vi "SteuerungWaermepumpe-altes FrontPanel_31.01.2017.vi"() -> ()   [LabVIEW 2015]
uses:
  <vilib>/DAQmx/read.llb/DAQmx Read (Analog 1D Wfm NChan NSamp).vi
  <vilib>/DAQmx/write.llb/DAQmx Write (Analog 1D Wfm NChan 1Samp).vi
  <vilib>/MakerHub/LINX/Public/Peripherals/Digital/Digital Write N Chans.vi
  <vilib>/MakerHub/LINX/Private/Local IO/LinxDigitalWrite.vi
  <vilib>/MakerHub/LINX/Public/Utilities/Check Channel.vi
  <vilib>/MakerHub/LINX/Private/Utilties/Generate Error.vi
  <vilib>/DAQmx/miscellaneous.llb/DAQmx Fill In Error Info.vi
  <vilib>/Utility/file.llb/Read Delimited Spreadsheet (DBL).vi
  <vilib>/MakerHub/LINX/LMH-LINX.lvlib
panel:
  in  "Keithley Messung?":bool
  in  "TI 21a SW °C":dbl=60.0 min=30.0 max=60.0
  in  "Öl-Regelung":bool
  out "Array 2":waveform(dbl)[](array[waveform])
  in  "Wartezeit 2":u32=500
  in  "Wartezeit 1":u32=9000
  out "Abscheider":cluster{dbl, dbl, dbl}(slide) scale=0.0..1.3
  in  "Rampe":bool=TRUE
  in  "Rampe rpm/s":dbl=1.0 min=1.0 max=100.0 step=1.0
  out "Rampe IW":dbl
  in  "reinitialize HD":bool
  in  "reinitialize Pumpe":bool
  out "ist an!":string
  in  "zusätzlicher Druck":dbl
  in  "PI05 SW":dbl format="%.2f"
  out "p_liq_mittel":dbl
  out "p_liq":dbl
  out "Schleifendauer":dbl format="%.5f"
  out "Mittelwert 2":dbl
  in  "Mittelwert HD":bool
  in  "Mittelwert Pumpe":bool
  out "Mittelwert":dbl
  in  "Xi / p_liq berechnung an":bool
  out "xi_r":dbl
  in  "Regler Senke":bool
  in  "reinitialize Senke":bool
  in  "TI35 SW":dbl=43.0 format="%.2f"
  in  "Drehzahl Bestätigung":bool
  in  "Drehzahl SW":dbl=1000.0 min=500.0 max=3000.0 step=1.0 format="%#_4g"
  out "Check":dbl format="%#_13g"
  in  "Regler Hochdruck":bool
  in  "PID Regelung Pumpe":bool
  in  "SW TI39":dbl
  out "Array":bool[](array[boolean])
  in  "LEDs 2":bool[](array[boolean])
  in  "Regelung HK":bool
  out "RV 30 zu":bool
  out "RV 30 auf":bool
  out "FI_Oel":dbl
  in  "RV 33":dbl(slide) scale=-1.0..1.0
  in  "tag":string
  out "Pumpenwerte":dbl[](array[numeric]) format="%.2f"
  out "Speichert!":bool
  out "Historie":string
  in  "Kommentar":string
  out "refnum out":refnum<file>
  in  "Identität!":string(combo)
  in  "Zeit X in Minuten":dbl(slide)=5.0 min=0.0 max=15.0 scale=5.0..15.0
  out "TI 21a Warnungen":dbl
  out "Leistung":dynamicdata(graph)
  out "TI 37":dbl
  in  "Programm stoppen!":bool
  out "%":sgl(slide) scale=0.0..100.0
  out "kalt":bool
  out "warm":bool
  out "?":T1(array[cluster]) {"?" format="%#.4g"; "Konzentration_reich" format="%#.4g"}
  in  "Mit EES vergleichen":bool
  in  "FI13 SW in l/min":dbl=3.0 min=3.0 max=20.0 step=0.10000000149011612
  out "COP_Oel":dbl
  out "Q-Oel kW":dbl format="%_4g"
  in  "Dateiname!":string
  in  "Comment":bool
  in  "Speichern":bool caption="Aktivieren"
  out "ZU     Ventilstellung 33     AUF":dbl(slide) scale=0.0..100.0 scale format="%.2f"
  in  "Regelventil 34":dbl(slide) min=0.0 max=100.0 step=0.009999999776482582 scale=0.0..100.0
  in  "Matlab":bool
  in  "?":T2(tab)
  out "?":dynamicdata(graph)
  out "?":waveform(dbl)(graph)
  out "?":dynamicdata(graph)
  out "PI 12":dbl format="%.2f"
  out "PI 11":dbl format="%.2f"
  out "Dichte":dbl format="%.5g"
  in  "Reset":bool
  out "Betriebszeit":cluster{"second":i32, "minute":i32, "hour":i32}
  out "Temperatur Ölprüfstand":dbl
  out "FI 13 kg/min":dbl
  in  "Messung\nFrequenzwandler":bool
  out "Magnetventil":bool
  out "Fl.Pumpe an":bool
  out "Temperatur Öl":bool
  out "COP":dbl format="%#_13g"
  out "Verdichteraktivität":cluster{"second":i32, "minute":i32, "hour":i32}
  out "Q-Entgaser kW":dbl format="%_4g"
  out "Warnungen":bool[](array[boolean])
  out "Status Komponenten":bool[](array[boolean])
  in  "Pumpen-Auto-Abschalt":bool=TRUE
  out "Q-Resorber kW":dbl format="%_4g"
  out "Stellung Expansionsventil":waveform(dbl)(graph)
  out "FI 35 l/min":dbl format="%#_13g"
  out "FI 38 l/min":dbl format="%#_13g"
  out "FI Oel l/min":dbl format="%#.3g"
  out "LI in l":dbl format="%#_4g"
  out "TI 39":dbl format="%#_3g"
  out "TI 38":dbl format="%#_3g"
  out "TI 36":dbl format="%#_3g"
  out "TI 35":dbl format="%#_3g"
  out "TI 33":dbl format="%#_3g"
  out "TI 32":dbl format="%#_3g"
  out "TI 34":dbl format="%#_3g"
  out "TI 21a":dbl format="%#_3g"
  out "TI 21":dbl format="%#_3g"
  out "TI 20":dbl format="%#_3g"
  out "TI 14a":dbl format="%#_3g"
  out "TI 14":dbl format="%#_3g"
  out "TI 13":dbl format="%#_3g"
  out "TI 12":dbl format="%#_3g"
  out "TI 11":dbl format="%#_3g"
  out "TI 10":dbl format="%#_3g"
  out "TI 09":dbl format="%#_3g"
  out "TI 08":dbl format="%#_3g"
  out "TI 07":dbl format="%#_3g"
  out "TI 06a":dbl format="%#_3g"
  out "TI 06":dbl format="%#_3g"
  out "TI 05":dbl format="%#_3g"
  out "TI 04":dbl format="%#_3g"
  out "TI 22":dbl format="%#_3g"
  out "TI 02":dbl format="%#_3g"
  out "TI 01":dbl format="%#_3g"
  out "Konzentration":dbl format="%#_5g"
  in  "Pumpensteuerung":dbl min=0.0 max=10.0 step=0.009999999776482582 format="%.2g"
  out "PI 08":dbl format="%.2f"
  out "PI 05":dbl format="%#.2f"
  out "PI 02":dbl format="%.2f"
  out "PI 04":dbl format="%.2f"
  out "PDI 8-9":dbl format="%.2f"
  out "PI 14":dbl format="%.2f"
  out "PI 01":dbl format="%.2f"
  out "ZU    Ventilstellung Exp.V     AUF":dbl(slide) scale=0.0..100.0 scale format="%#.1f"
  in  "Exp.V":dbl(slide)=3.0 min=0.0 max=100.0 step=1.0 scale=0.0..100.0 scale format="%#.0f"
  out "ZU    Ventilstellung 14      AUF":dbl(slide) caption="Auf    Ventilstellung 14      Zu" scale=0.0..100.0 scale format="%#.2f"
  in  "Regelventil 36":dbl(slide) min=0.0 max=100.0 step=0.009999999776482582 scale=0.0..100.0 scale format="%#.0f"
  out "ZU  Ventilstellung 35  AUF":dbl(slide) scale=0.0..100.0 scale format="%.2f"
  in  "Regelventil 35":dbl(slide) min=0.0 max=100.0 step=0.009999999776482582 scale=0.0..100.0 scale format="%#.3g"
  out "ZU     Ventilstellung 39     AUF":dbl(slide) scale=0.0..100.0 scale format="%.2f"
  in  "Regelventil 39":dbl(slide)=100.0 min=0.0 max=100.0 step=0.009999999776482582 scale=0.0..100.0
  out "FI 13 l/min":dbl format="%.2f"
  out "FI 07 l/min":dbl format="%.2f"
  out "LI in m":dbl format="%.2f"
  out "PDI 5-6":dbl format="%.4f"
  out "PI 07":dbl format="%.2f"
  out "Druckverhältnis":dbl
  out "Drehzahl":dbl
  out "Drehmoment":dbl
  out "Frequenz":dbl
  out "Leistung":dbl
  out "Durchfluss":waveform(dbl)[](graph)
  in  "Tab Control Temperaturen":T3(tab)
  out "Temperatur Reich":waveform(dbl)[](graph)
  out "Temperatur Arm":waveform(dbl)[](graph)
  out "Temperatur Öl":waveform(dbl)[](graph)
  out "Temperatur Senke/Quelle":waveform(dbl)[](graph)
  out "Druck":waveform(dbl)[](graph)
  out "Druckzustand":bool caption="Zu viel Druck !!!"
  # "Öltemperatur"
  # "Resorber"
  # "Entgaser"
  # "Druckverhältnis"
  # "ExpV"
  # "Verdichter an"
  # "iWÜ"
  # "Magnetventil"
  # "RV 39"
  # "Leer"
  # "RV 33"
  # "RV 35"
  # "RV 34"
  # "Pumpe an"
  # "Ölabscheider"
  # "2"
  # "1"
  # "RV 30"
  # "Verdichter"
  # "Pumpe"
  # "Leistung"
  # "kW"
  # "Speed"
  # "rpm"
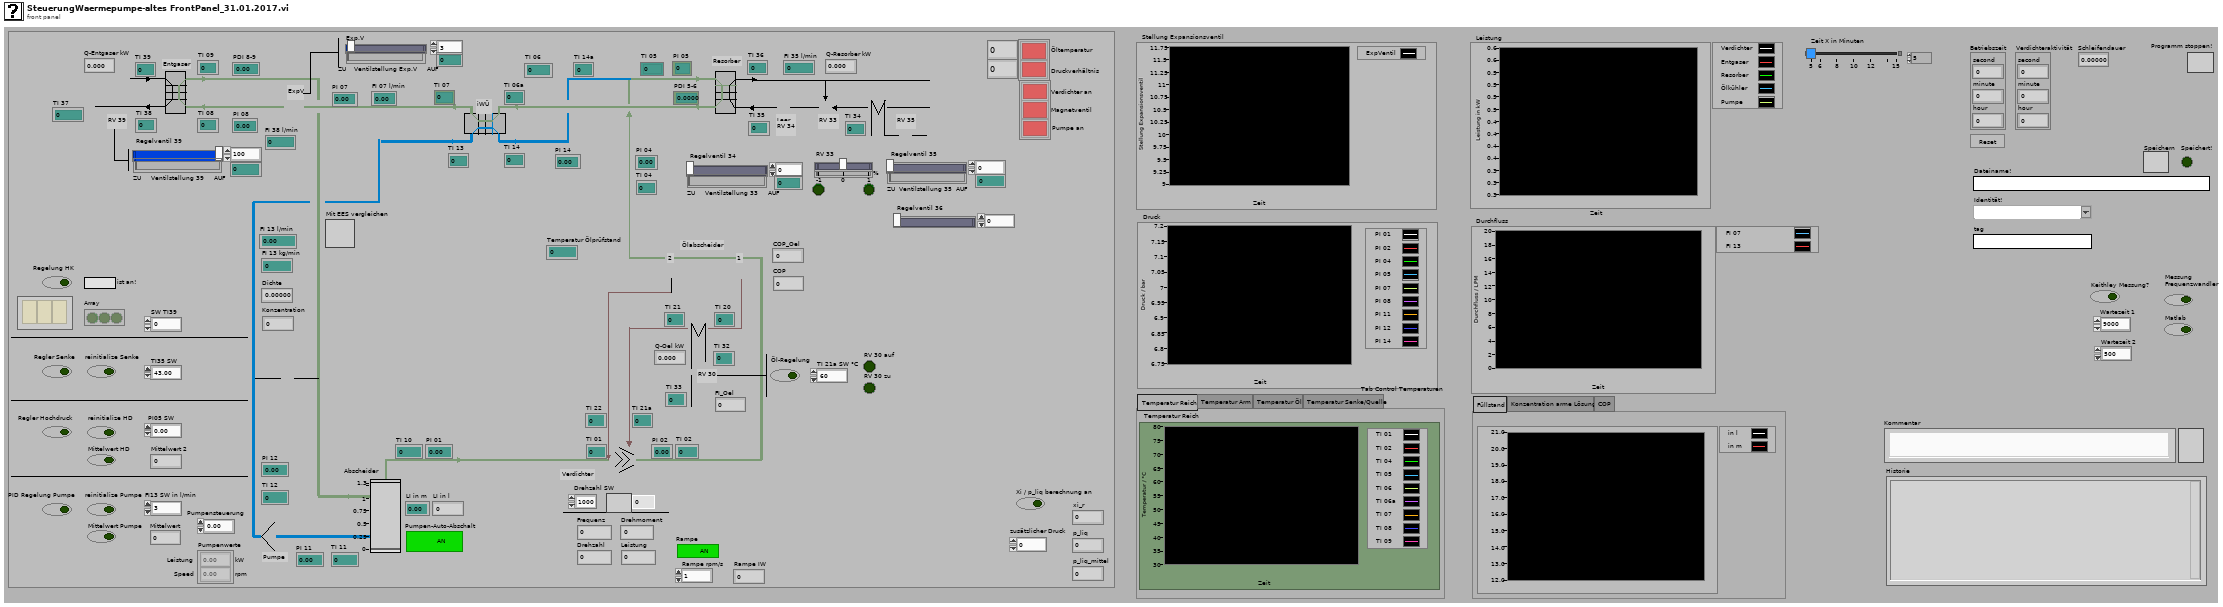
[diagram p1: front panel]
types:
  T1 = cluster{dbl, "Konzentration_reich":dbl, "String":string, bool}[]
  T2 = enum32{"Füllstand", "Konzentration arme Lösung", "COP"}
  T3 = enum32{"Temperatur Reich", "Temperatur Arm", "Temperatur Öl", "Temperatur Senke/Quelle"}
  T4 = enum8{"Enabled", "Disabled", "Disabled and Grayed Out"}
  T5 = typedef "LMH-LINX.lvlib/LINX Ref.ctl" = cluster{"IO":T6, "Interface":T7, "LINX Device Config":T8}
  T6 = typedef "LMH-LINX.lvlib/Platform.ctl" = enum16{"Remote", "Local"}
  T7 = typedef "LMH-LINX.lvlib/Interface.ctl" = enum16{"Serial", "TCP"}
  T8 = typedef "LMH-LINX.lvlib/Device.lvlib/LINX Device Config.ctl" = cluster{"Interface":T7, "COM Port":refnum<visa-resource-name>, "TCP Configuration":T9, "Device Family":u8, "Device ID":u8, "Device Name":string, "TCP Ref":refnum<k5>, "Channels":T10}
  T9 = typedef "LMH-LINX.lvlib/Device.lvlib/TCP Config.ctl" = cluster{"IP Address":string, "Port":u16}
  T10 = typedef "LMH-LINX.lvlib/Channels.ctl" = cluster{"DI":u8[], "DO":u8[], "AI":u8[], "AO":u8[], "PWM":u8[], "QE":u8[], "UART":u8[], "I2C 2":u8[], "SPI":u8[], "CAN":u8[], "Servo":u8[], "AI Ref (V)":dbl, "AI Resolution (Bits)":u8, "AO Ref (V)":dbl, "AO Resolution (Bits)":u8}
  T11 = enum16{"open", "replace", "create", "open or create", "replace or create", "replace or create with confirmation"}
  T12 = cluster{"Array[0]":dbl, "Array[1]":dbl, "Array[2]":dbl}
  T13 = cluster{"Array[0]":sgl, "Array[1]":sgl, "Array[2]":sgl}
  T14 = cluster{"Numeric":dbl, "Konzentration_reich":dbl, "String":string, bool}[]
  T15 = typedef "LVDateTimeRec.ctl" = cluster{"fractional second":dbl, "second":i32, "minute":i32, "hour":i32, "day of month":i32, "month":i32, "year":i32, "day of week":i32, "day of year":i32, "DST":i32}
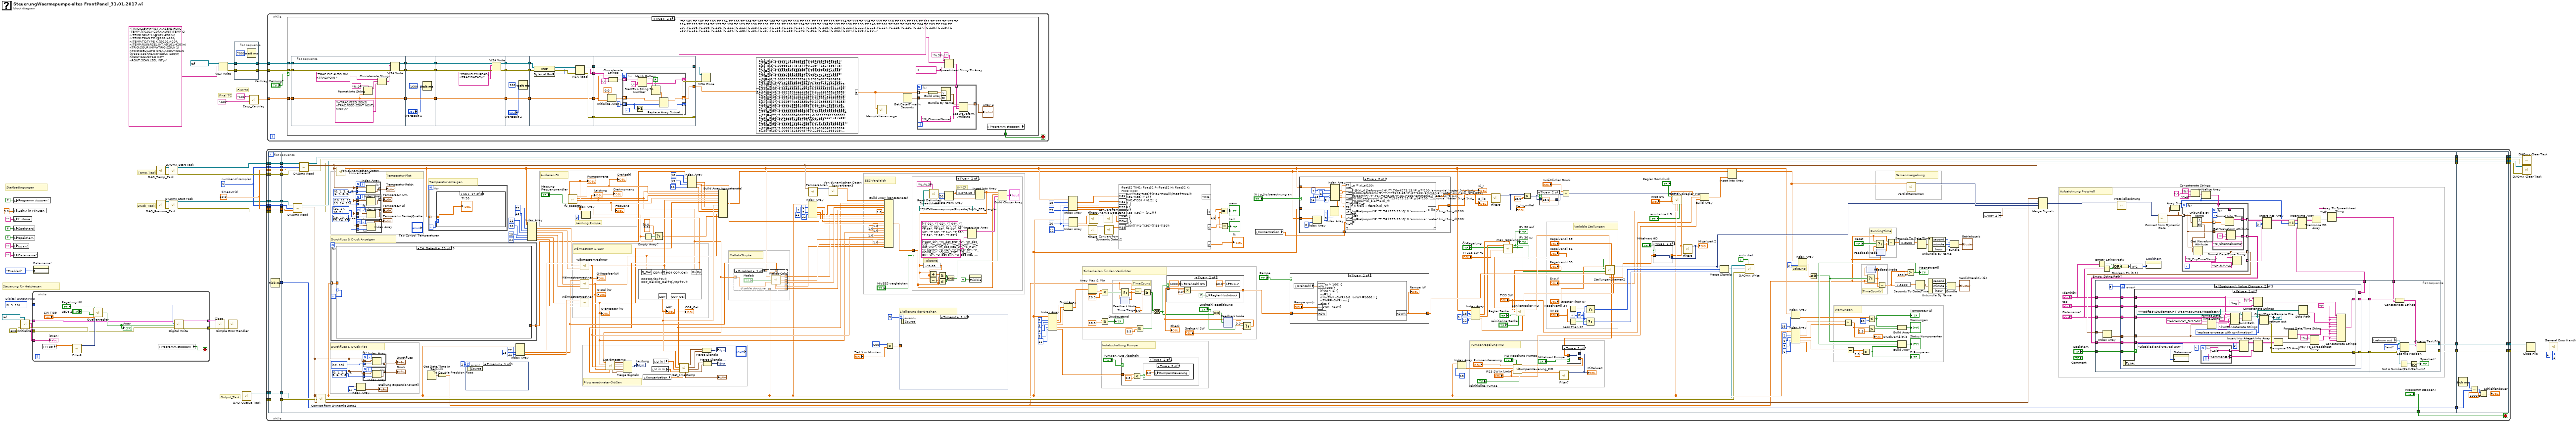
[diagram p0: block diagram]
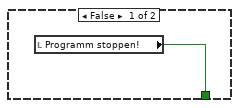
[diagram p2: hidden frame]
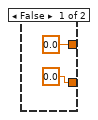
[diagram p8: hidden frame]
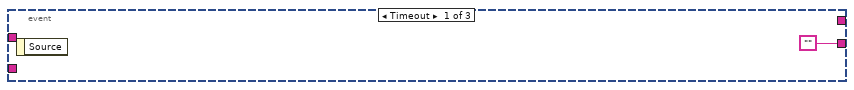
[diagram p10: hidden frame]
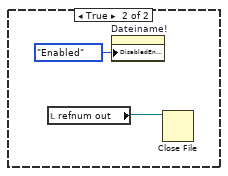
[diagram p11: hidden frame]
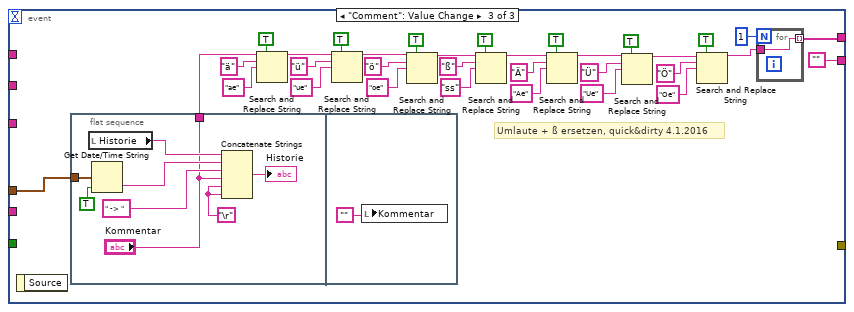
[diagram p12: hidden frame]
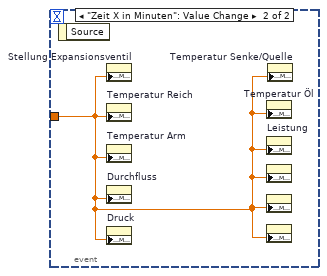
[diagram p13: hidden frame]
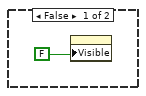
[diagram p14: hidden frame]
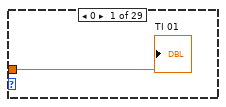
[diagram p17: hidden frame]
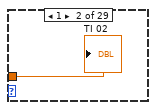
[diagram p18: hidden frame]
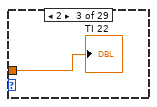
[diagram p19: hidden frame]
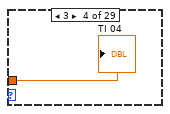
[diagram p20: hidden frame]
diagram:
  w19 = 10.0  # timeout (s)
  w18 = 1  # number of samples
  w31 = i32[] [8, 9, 10]  # Digital Output PIns
  # "Final TC"
  # "First TC"
  # "Output_Task"
  # "Druck_Task"
  # "Temp_Task"
  # "Steuerung für Heizkerzen"
  # "Startbedingungen"
  n1 = local write "Programm stoppen!"(FALSE ("Programm stoppen!")) -> ()
  n2 = local write "Zeit X in Minuten"(5.0 ("Zeit X in Minuten")) -> ()
  n3 = local write "Historie"("") -> ()
  n4 = local write "Speichert!"(FALSE ("Speichert!")) -> ()
  n5 = local write "Speichern"(FALSE ("Speichern")) -> ()
  n6 = local write "ist an!"("") -> ()
  n7 = local write "Dateiname!"("") -> ()
  n8 = call <vilib>:"Initialize.vi"("Serial Port"=refnum<visa-resource-name> "COM4", "Error In"=errorcluster {"status"=FALSE, "code"=0, "source"=""}) -> ("Error Out"=w32:errorcluster, "Device Name"=w29:string, "LINX Resource"=w35:T5)  [unwired: 7 in]
  n9 = while {
    tunnel: w35 -> [w50]
    tunnel: [w60] -> w34
    tunnel: [w59] -> w33
    tunnel: w32 -> [w49]
    tunnel: w31 -> [w58]
    tunnel: w29 -> [w48]
    stop <- w57 stop-if-true
    n10 = local read "TI 39"() -> (w51:dbl)
    n11 = call "Filter6"("Signal"=w51) -> ("Filtered Signal"=w52:dynamicdata)  [unwired: 9 in, 1 out]
    n12 = call "Quellenregler.vi"("Regelung Quelle"="Regelung HK", "TI 38 IW °C"=w52, "LEDs"="LEDs 2", "TI 38 SW °C"="SW TI39") -> ("Kerzen von Regler"=w54:bool[])  [unwired: 3 in, 1 out]
    "Array" <- w54
    n13 = local read "Programm stoppen!"() -> (w57:bool)
    n14 = call-poly <vilib>:"Digital Write.vi"("Error In"=w49, "Values"=w54, "DO Channels"=w58, "LINX Resource"=w50) -> ("Error Out"=w59:errorcluster, "LINX Resource"=w60:T5)  [unwired: 6 in]
    "ist an!" <- w48
  }
  n15 = property on="Dateiname!" class="Str"("DisabledEnum"=T4."Enabled" ("Disabled")) -> ()  [unwired: 2 in, 2 out]
  n16 = call "DAQ_Pressure_Task.vi"() -> ("error out"=w23:errorcluster, "task out"=w24:refnum<k21>)  [unwired: 10 in]
  n17 = call "DAQ_Temp_Task.vi"() -> ("error out"=w25:errorcluster, "task out"=w26:refnum<k21>)  [unwired: 10 in]
  n18 = call <vilib>:"DAQmx Start Task.vi"("task/channels in"=w24, "error in"=w23) -> ("task out"=w17:refnum<k21>, "error out"=w20:errorcluster)  [unwired: 12 in]
  n19 = call <vilib>:"DAQmx Start Task.vi"("task/channels in"=w26, "error in"=w25) -> ("task out"=w21:refnum<k21>, "error out"=w22:errorcluster)  [unwired: 12 in]
  n20 = call <vilib>:"Close.vi"("Error In"=w33, "LINX Resource"=w34) -> ("Error Out"=w36:errorcluster)  [unwired: 9 in]
  n21 = VISA Write(VISA resource name=refnum<visa-resource-name> "COM3", write buffer="TRAC:CLE\n\n*RST\n\nSENS:FUNC 'TEMP',(@101:420)\n\nUNIT:TEMP C\n:TEMP:NPLC 1,(@101:420)\n\n:TEMP:TRAN TC,(@101:420)\n:TEMP:TC:TYPE K,(@101:420)\n:TEMP:RJUN:RSEL INT,(@101:420)\n\nTRIG:SOUR IMM\nTRIG:COUN 1\nTRIG:DEL:AUTO ON\n\nROUT:SCAN  (@101:420)\nSAMP:COUN 120\n\nROUT:SCAN:TSO IMM\nROUT:SCAN:LSEL INT\n") -> (VISA resource name out=w5:refnum<visa-resource-name>, error out=w6:errorcluster)  [unwired: 1 in, 1 out]
  n22 = call <vilib>:"Simple Error Handler.vi"("error in (no error)"=w36) -> ()  [unwired: 4 in, 5 out]
  n23 = flat-sequence {
    tunnel: w6 -> [w63]
    tunnel: [w63] -> w3
    tunnel: w5 -> [w61]
    tunnel: [w61] -> w4
    frame #0 {
      n24 = Wait (ms)(milliseconds to wait=u32 7000 ("Zu wartende ms")) -> ()  [unwired: 1 out]
    }
  }
  n25 = call "DAQ_Output_Task.vi"() -> ("error out"=w11:errorcluster, "task out"=w12:refnum<k21>)  [unwired: 10 in]
  n26 = call "Easy_Keithley.vi"("Final Thermocouple ID# (String)"="420", "First Thermocouple ID# (String)"="101") -> ("Number of Thermocouples"=w7:dbl)  [unwired: 8 in, 1 out]
  n27 = while {
    tunnel: [w98] -> w41
    tunnel: [w97] -> w40
    tunnel: w22 -> [w91]
    tunnel: w19 -> [w89]
    tunnel: w21 -> [w86]
    tunnel: w18 -> [w84]
    tunnel: w20 -> [w82]
    tunnel: w19 -> [w81]
    tunnel: w18 -> [w79]
    tunnel: w17 -> [w77]
    tunnel: [w73] -> w16
    tunnel: [w72] -> w15
    tunnel: [w70] -> w14
    tunnel: [w68] -> w13
    tunnel: w12 -> [w67]
    tunnel: w11 -> [w64]
    stop <- w96 stop-if-true
    n28 = flat-sequence {
      tunnel: [w109] -> w92
      tunnel: w91 -> [w108]
      tunnel: [w108] -> w90
      tunnel: w89 -> [w107]
      tunnel: [w107] -> w88
      tunnel: w86 -> [w106]
      tunnel: [w106] -> w87
      tunnel: [w105] -> w85
      tunnel: w84 -> [w105]
      tunnel: [w104] -> w83
      tunnel: w82 -> [w104]
      tunnel: w81 -> [w103]
      tunnel: [w103] -> w80
      tunnel: w79 -> [w102]
      tunnel: [w102] -> w78
      tunnel: w77 -> [w101]
      tunnel: [w101] -> w76
      tunnel: w67 -> [w100]
      tunnel: [w100] -> w66
      tunnel: [w99] -> w65
      tunnel: w64 -> [w99]
      tunnel: ["Programm stoppen!"] -> w96
      tunnel: [w333] -> w95
      tunnel: [w332] -> w94
      tunnel: [w141] -> w93
      tunnel: w92 -> [w141]
      tunnel: w90 -> [w176]
      tunnel: w88 -> [w175]
      tunnel: w87 -> [w174]
      tunnel: w85 -> [w173]
      tunnel: w83 -> [w172]
      tunnel: w80 -> [w171]
      tunnel: w78 -> [w170]
      tunnel: w76 -> [w169]
      tunnel: [w168] -> w75
      tunnel: [w167] -> w74
      tunnel: [w166] -> w71
      tunnel: [w165] -> w69
      tunnel: w66 -> [w163]
      tunnel: w65 -> [w162]
      tunnel: [w742] -> w97
      tunnel: [w743] -> w98
      tunnel: w95 -> [w743]
      tunnel: w94 -> [w742]
      tunnel: w93 -> [w740]
      tunnel: w75 -> [w735]
      tunnel: w74 -> [w736]
      tunnel: [w736] -> w73
      tunnel: [w735] -> w72
      tunnel: w71 -> [w734]
      tunnel: [w734] -> w70
      tunnel: w69 -> [w733]
      tunnel: [w733] -> w68
      frame #0 {
        n29 = Tick Count (ms)() -> (millisecond timer value=w109:u32)
      }
      frame #1 {
        w143 = 8.0  # Time Target
        w164 = TRUE  # auto start
        w353 = sgl 1.0
        w366 = 22
        w371 = 20
        w397 = -4
        w398 = 0
        # "RunningTime"
        # "TimeCountV"
        # "TimeCount"
        # "Sicherheiten für den Verdichter"
        # "Pumpenregelung PID"
        # "Skalierung der Graphen"
        # "Leistung Pumpe"
        # "Leistung"
        # "Durchfluss & Druck Anzeigen"
        # "Temperatur Anzeigen"
        # "Plots errechneter Größen"
        # "EES-Vergleich"
        # "Matlab-Skripte"
        # "Warnungen"
        # "Namensvergebung"
        # "Wärmestrom & COP"
        # "Notabschaltung Pumpe"
        # "Auslesen FU"
        # "Durchfluss & Druck Plot"
        # "Temperatur Plot"
        # "Aufzeichnung Protokoll"
        # "Variable Stellungen"
        n30 = call-poly <vilib>:"DAQmx Read.vi"("task/channels in"=w169, "number of samples per channel"=w170, "timeout"=w171, "error in"=w172) -> ("task out"=w168:refnum<k21>, "data"=w178:waveform(dbl)[], "error out"=w165:errorcluster)  [unwired: 9 in]
        n31 = call-poly <vilib>:"DAQmx Read.vi"("task/channels in"=w174, "number of samples per channel"=w173, "timeout"=w175, "error in"=w176) -> ("task out"=w167:refnum<k21>, "data"=w177:waveform(dbl)[], "error out"=w166:errorcluster)  [unwired: 9 in]
        n32 = call "Convert from Dynamic Data2"("Dynamic Data Type"=w178) -> ("Array"=w183:dbl[])  [unwired: 3 in]
        n33 = for {
          tunnel: w183 -> [w681] mode=indexing
          tunnel: [w680] -> w188 mode=indexing
          i -> [w682]
          n34 = case shown="24, Default" w682 {
            tunnel: w681 -> [w683 w684 w685 w686 w687 w688 w689 w690 w691 w692 w693 w702 w714 w717 w718 w719 w720 w721 w724 w728 w729 w730 w731 w732 _]
            tunnel: [_ _ _ _ _ _ _ _ _ _ _ w694 _ _ _ _ _ _ w722 w726 _ _ _ _ _] -> w680
            frame 0 {
              "PI 01" <- w683
            }
            frame 1 {
              "PI 02" <- w684
            }
            frame 2 {
              "PI 04" <- w685
            }
            frame 3 {
              "PI 05" <- w686
            }
            frame 4 {
              "PI 07" <- w687
            }
            frame 5 {
              "PI 08" <- w688
            }
            frame 6 {
              "PI 11" <- w689
            }
            frame 7 {
              "PI 12" <- w690
            }
            frame 8 {
              "PI 14" <- w691
            }
            frame 9 {
              "PDI 5-6" <- w692
            }
            frame 10 {
              "PDI 8-9" <- w693
            }
            frame 11 {
              n35 = call "Filter3"("Signal"=w702) -> ("Filtered Signal"=w700:dynamicdata)  [unwired: 9 in, 1 out]
              n36 = Greater?(x=w702, y=0.3) -> (0:w697:bool)
              n37 = case shown="False" w697 {
                tunnel: w702 -> [_ w713]
                tunnel: [0.0 w713] -> w705
                frame False {
                }
                frame True {
                }
              }
              n38 = call "Convert from Dynamic Data6"("Dynamic Data Type"=w700) -> ("Scalar"=w699:dbl)  [unwired: 3 in]
              n39 = Multiply(x=w699, y=10.0) -> (x*y=w701:dbl)
              n40 = Greater?(x=w702, y=0.4) -> (0:w698:bool)
              n41 = formula code="float64 y; float64 Vu; /*Vu: Volumen schmaler Zylinder+Fuellstandsmesser*/\nVu=10;  /* 10 Liter */\n\nif (x<=10.25) \ny=(x-1)*pi*(0.536**2+0.32**2);\nelse\ny=Vu+(x-10.25)*pi*(1.584**2+0.32**2);"("x"=w701) -> ("y"=w694:dbl)
              "LI in l" <- w694
              n42 = case shown="False" w698 {
                tunnel: w702 -> [_ w711]
                tunnel: [0.0 w711] -> w704
                frame False {
                }
                frame True {
                }
              }
              n43 = Merge Signals(w702, w705, w704) -> (w706:dynamicdata)
              n44 = call "Convert from Dynamic Data3"("Dynamic Data Type"=w706) -> ("Array"=w709:dbl[])  [unwired: 3 in]
              n45 = Array To Cluster(array=w709) -> (cluster=w696:T12)
              n46 = To Single Precision Float(number=w696) -> (single precision float=→"Abscheider":T13)
              "LI in m" <- w702
            }
            frame 12 {
              "FI 07 l/min" <- w714
            }
            frame 13 {
              n47 = local read "Dichte"() -> (w716:dbl)
              n48 = Multiply(x=w717, y=w716) -> (x*y=→"FI 13 kg/min":dbl)
              "FI 13 l/min" <- w717
            }
            frame 14 {
              "ZU     Ventilstellung 39     AUF" <- w718
              "ZU     Ventilstellung 33     AUF" <- w718
            }
            frame 15 {
              "ZU  Ventilstellung 35  AUF" <- w719
            }
            frame 16 {
              # "RV14 ist entfernt"
              "ZU    Ventilstellung 14      AUF" <- w720
            }
            frame 17 {
              "ZU    Ventilstellung Exp.V     AUF" <- w721
            }
            frame 18 {
              n49 = call "Filter"("Signal"=w724) -> ("Filtered Signal"=w723:dynamicdata)  [unwired: 9 in, 1 out]
              n50 = call "Convert from Dynamic Data4"("Dynamic Data Type"=w723) -> ("Scalar"=w725:dbl)  [unwired: 3 in]
              n51 = formula code="float64 D;\nD=9.375*StromDichte+0.7125;\nD=floor(D*100000)/100000;"("StromDichte"=w725) -> ("D"=w722:dbl)
              "Dichte" <- w722
            }
            frame 19 {
              n52 = call "Filter2"("Signal"=w728) -> ("Filtered Signal"=w727:dynamicdata)  [unwired: 9 in, 1 out]
              n53 = To Double Precision Float(number=w727) -> (double precision float=w726:dbl)
              "Konzentration" <- w726
            }
            frame 20 {
              "FI Oel l/min" <- w729
            }
            frame 21 {
              "FI 38 l/min" <- w730
            }
            frame 22 {
              "FI 35 l/min" <- w731
            }
            frame 23 {
              "FI_Oel" <- w732
            }
            frame 24, Default {
            }
          }
        }
        n54 = call "Von dynamischen Daten konvertieren2"("Dynamic Data Type"=w177) -> ("Array"=w126:dbl[])  [unwired: 3 in]
        n55 = for {
          tunnel: i32[] [0, 1, 3, 4, 5, 6, 7, 8, 9] -> [w495] mode=indexing
          tunnel: w177 -> [w494]
          tunnel: [w493] -> w269 mode=indexing
          n56 = Index Array(array=w494, index=w495) -> (element=w493:waveform(dbl))
        }
        "Temperatur Reich" <- w269
        n57 = for {
          tunnel: i32[] [10, 11, 12, 13, 14, 15] -> [w492] mode=indexing
          tunnel: w177 -> [w491]
          tunnel: [w490] -> w270 mode=indexing
          n58 = Index Array(array=w491, index=w492) -> (element=w490:waveform(dbl))
        }
        "Temperatur Arm" <- w270
        n59 = for {
          tunnel: i32[] [16, 17, 18, 2] -> [w489] mode=indexing
          tunnel: w177 -> [w488]
          tunnel: [w487] -> w271 mode=indexing
          n60 = Index Array(array=w488, index=w489) -> (element=w487:waveform(dbl))
        }
        "Temperatur Öl" <- w271
        n61 = Index Array(array=w178, index=17) -> (element=→"Stellung Expansionsventil":waveform(dbl))
        n62 = for {
          tunnel: i32[] [19, 20, 21, 22, 23, 24, 25] -> [w486] mode=indexing
          tunnel: w177 -> [w485]
          tunnel: [w484] -> w272 mode=indexing
          n63 = Index Array(array=w485, index=w486) -> (element=w484:waveform(dbl))
        }
        "Temperatur Senke/Quelle" <- w272
        n64 = for {
          tunnel: [w480] -> w267 mode=indexing
          tunnel: w178 -> [w479]
          tunnel: i32[] [0, 1, 2, 3, 4, 5, 6, 7, 8] -> [w478] mode=indexing
          n65 = Index Array(array=w479, index=w478) -> (element=w480:waveform(dbl))
        }
        "Druck" <- w267
        n66 = for {
          tunnel: [w483] -> w268 mode=indexing
          tunnel: w178 -> [w482]
          tunnel: i32[] [12, 13] -> [w481] mode=indexing
          n67 = Index Array(array=w482, index=w481) -> (element=w483:waveform(dbl))
        }
        "Durchfluss" <- w268
        n68 = Get Date/Time In Seconds() -> (seconds since 1Jan1904=w140:timestamp)
        n69 = for {
          tunnel: w126 -> [w650] mode=indexing
          i -> [w651]
          n70 = case shown="16" w651 {
            tunnel: w650 -> [w652 w653 w654 w655 w656 w657 w658 w659 w660 w661 w662 w663 w664 w665 w666 w667 w668 w669 w670 w671 w672 w673 w674 w675 w676 w677 w678 w679 _]
            frame 0 {
              "TI 01" <- w652
            }
            frame 1 {
              "TI 02" <- w653
            }
            frame 2 {
              "TI 22" <- w654
            }
            frame 3 {
              "TI 04" <- w655
            }
            frame 4 {
              "TI 05" <- w656
            }
            frame 5 {
              "TI 06" <- w657
            }
            frame 6 {
              "TI 06a" <- w658
            }
            frame 7 {
              "TI 07" <- w659
            }
            frame 8 {
              "TI 08" <- w660
            }
            frame 9 {
              "TI 09" <- w661
            }
            frame 10 {
              "TI 10" <- w662
            }
            frame 11 {
              "TI 11" <- w663
            }
            frame 12 {
              "TI 12" <- w664
            }
            frame 13 {
              "TI 13" <- w665
            }
            frame 14 {
              "TI 14" <- w666
            }
            frame 15 {
              "TI 14a" <- w667
            }
            frame 16 {
              "TI 20" <- w668
            }
            frame 17 {
              "TI 21" <- w669
            }
            frame 18 {
              "TI 21a" <- w670
              "TI 21a Warnungen" <- w670
            }
            frame 19 {
              # "Check T_Heater"
              "TI 34" <- w671
            }
            frame 20 {
              "TI 32" <- w672
            }
            frame 21 {
              "TI 33" <- w673
            }
            frame 22 {
              "TI 35" <- w674
            }
            frame 23 {
              "TI 36" <- w675
            }
            frame 24 {
              "TI 38" <- w676
            }
            frame 25 {
              "TI 39" <- w677
            }
            frame 26 {
              "Temperatur Ölprüfstand" <- w678
            }
            frame 27 {
              "TI 37" <- w679
            }
            frame 28, Default {
            }
          }
        }
        n71 = To Double Precision Float(number=w140) -> (double precision float=w128:dbl)
        n72 = event shown="[0] Timeout" {
          selector: _ -> [_]
          dyn-events: _ -> [_]
          timeout: 2 -> [_]
          event Timeout {
            n73 = event-data() -> ()  [unwired: 1 in, 1 out]
          }
        }
        n74 = Index Array(array=w183, index #1=22 ("index"), index #2=23 ("index"), index #3=21 ("index")) -> (element #1=w302:dbl, element #2=w278:dbl, element #3=w301:dbl)
        n75 = Index Array(array=w126, index #1=22 ("index"), index #2=23 ("index"), index #3=21 ("index"), index #4=20 ("index"), index #5=25 ("index"), index #6=24 ("index")) -> (element #1=w300:dbl, element #2=w299:dbl, element #3=w298:dbl, element #4=w297:dbl, element #5=w296:dbl, element #6=w295:dbl)
        n76 = call "fu_gesamt.vi"("Boolean"="Messung\nFrequenzwandler") -> ("Frequenz"=w290:dbl, "Drehmoment"=w291:dbl, "Leistung"=w151:dbl, "Drehzahl"=w292:dbl, "Scaled"=w153:dbl[])  [unwired: 6 in]
        "Leistung" <- w151
        "Frequenz" <- w290
        "Drehmoment" <- w291
        "Drehzahl" <- w292
        "Pumpenwerte" <- w153
        n77 = call "Wärmestromrechner.vi"("Taus"=w299, "Tein"=w300, "Massenstrom"=w302) -> ("Wärmestrom Q"=w202:dbl)  [unwired: 2 in]
        "Q-Resorber kW" <- w202
        n78 = call "Wärmestromrechner.vi"("Taus"=w297, "Tein"=w298, "Massenstrom"=w278) -> ("Wärmestrom Q"=w189:dbl)  [unwired: 2 in]
        "Q-Oel kW" <- w189
        n79 = call "Wärmestromrechner.vi"("Taus"=w295, "Tein"=w296, "Massenstrom"=w301) -> ("Wärmestrom Q"=w201:dbl)  [unwired: 2 in]
        "Q-Entgaser kW" <- w201
        n80 = Index Array(array=w153, index=0) -> (element=w203:dbl)
        n81 = call "Set_timestamp.vi"("Eingang 5"=w203, "Eingang 4"=w189, "Eingang 3"=w202, "Eingang 2"=w201, "Eingang"=w151) -> ("Ausgang 4"=w199:waveform(dbl), "Ausgang 3"=w198:waveform(dbl), "Ausgang 2"=w197:waveform(dbl), "Ausgang"=w196:waveform(dbl), "Ausgang 5"=w200:waveform(dbl))  [unwired: 2 in]
        n82 = Merge Signals(w196, w197, w198, w199, w200) -> (→"Leistung":dynamicdata)
        n83 = formula code="float64 COP; float64 COP_Oel;\n\nCOP=Q/(Pp+Pv);\nCOP_Oel=(Q_Oel+Q)/(Pp+Pv);"("Pv"=w151, "Q"=w202, "Pp"=w203, "Q_Oel"=w189) -> ("COP"=w211:dbl, "COP_Oel"=w210:dbl)
        "COP" <- w211
        "COP_Oel" <- w210
        n84 = local read "Konzentration"() -> (w215:dbl)
        n85 = Empty Array?(array=w153) -> (empty?=w155:bool)
        n86 = local read "LI in m"() -> (w213:dbl)
        n87 = local read "LI in l"() -> (w212:dbl)
        n88 = Select(t=dbl[] [0.0, 0.0], s=w155, f=w153) -> (s? t:f=w152:dbl[])
        n89 = call "Set_timestamp.vi"("Eingang 5"=w215, "Eingang 4"=w213, "Eingang 3"=w212, "Eingang 2"=w211, "Eingang"=w210) -> ("Ausgang 4"=w208:waveform(dbl), "Ausgang 3"=w207:waveform(dbl), "Ausgang 2"=w205:waveform(dbl), "Ausgang"=w204:waveform(dbl), "Ausgang 5"=→"?":waveform(dbl))  [unwired: 2 in]
        n90 = Index Array(array=w188, index #1=18 ("index"), index #2=19 ("index"), index #3=11 ("index")) -> (element #1=w190:dbl, element #2=w187:dbl, element #3=w191:dbl)
        n91 = Merge Signals(w204, w205) -> (→"?":dynamicdata)
        n92 = Merge Signals(w207, w208) -> (→"?":dynamicdata)
        n93 = Build Array (concatenate)(w151, w292, w291, w290, w202, w201, w211, w190, w187, w191, w189, w152) -> (w125:dbl[])
        n94 = disable-structure shown="Disabled" {
          disable-tunnel: [w440 _] -> w394
          disable-tunnel: [w439 _] -> w383
          disable-tunnel: [w438 _] -> w372
          disable-tunnel: [w437 _] -> w294
          disable-tunnel: [w436 _] -> w289
          disable-tunnel: w278 -> [w435 _]
          disable-tunnel: w151 -> [w434 _]
          disable-tunnel: w183 -> [w433 _]
          disable-tunnel: w126 -> [w432 _]
          frame Disabled {
            n95 = call "Matlab-Calc.vi"("Temp-Array"=w432, "Matlab?"="Matlab", "Leistung"=w434, "Druck-Array"=w433, "FI Öl"=w435) -> ("m_reich [g/s]"=w439:dbl, "Konzentration_reich"=w436:dbl, "m_arm [g/s]"=w440:dbl, "Dampfmassenstrom [g/s]"=w437:dbl, "Dampfmassenanteil"=w438:dbl)  [unwired: 3 in, 7 out]
          }
          frame Enabled {
          }
        }
        n96 = Index Array(array=w183, index #1=0 ("index"), index #2=1 ("index"), index #3=2 ("index"), index #4=21 ("index"), index #5=22 ("index")) -> (element #1=w377:dbl, element #2=w378:dbl, element #3=w379:dbl, element #4=w376:dbl, element #5=w374:dbl)
        n97 = call "Temperaturen"("Signals"=w177) -> ("Signal Out"=w384:dynamicdata)  [unwired: 9 in, 1 out]
        n98 = call "Von dynamischen Daten konvertieren3"("Dynamic Data Type"=w384) -> ("Array"=w385:dbl[])  [unwired: 3 in]
        n99 = Build Array (concatenate)(w385, w210, w376, w394, w383, 1.0 ("element"), w294, w374, w379, w378, w377, 1.0 ("element"), 1.0 ("element"), 1.0 ("element"), w201, 1.0 ("element"), w202, w372, 1.0 ("element"), w187, w289) -> (w386:dbl[])
        n100 = Multiply(x=600, y="Zeit X in Minuten") -> (x*y=w345:dbl)
        n101 = event shown="[0] Timeout" {
          selector: _ -> [_ _]
          dyn-events: _ -> [_ _]
          timeout: 5 -> [_ _]
          tunnel: w345 -> [_ w624]
          event Timeout {
            n102 = event-data() -> ()  [unwired: 1 in, 1 out]
          }
          event "Zeit X in Minuten": Value Change {
            n103 = event-data() -> ()  [unwired: 1 in, 1 out]
            n104 = property on="Stellung Expansionsventil" class="WFChart (strict)"("XScale.Maximum"=w624) -> ()  [unwired: 2 in, 2 out]
            n105 = property on="Temperatur Reich" class="WFChart (strict)"("XScale.Maximum"=w624) -> ()  [unwired: 2 in, 2 out]
            n106 = property on="Temperatur Arm" class="WFChart (strict)"("XScale.Maximum"=w624) -> ()  [unwired: 2 in, 2 out]
            n107 = property on="Durchfluss" class="WFChart (strict)"("XScale.Maximum"=w624) -> ()  [unwired: 2 in, 2 out]
            n108 = property on="Druck" class="WFChart (strict)"("XScale.Maximum"=w624) -> ()  [unwired: 2 in, 2 out]
            n109 = property on="Temperatur Öl" class="WFChart (strict)"("XScale.Maximum"=w624) -> ()  [unwired: 2 in, 2 out]
            n110 = property on="Leistung" class="WFChart (strict)"("XScale.Maximum"=w624) -> ()  [unwired: 2 in, 2 out]
            n111 = property class="WFChart (strict)"("XScale.Maximum"=w624) -> ()  [unwired: 2 in, 2 out]
            n112 = property class="WFChart (strict)"("XScale.Maximum"=w624) -> ()  [unwired: 2 in, 2 out]
            n113 = property class="WFChart (strict)"("XScale.Maximum"=w624) -> ()  [unwired: 2 in, 2 out]
            n114 = property on="Temperatur Senke/Quelle" class="WFChart (strict)"("XScale.Maximum"=w624) -> ()  [unwired: 2 in, 2 out]
          }
        }
        n115 = case shown="True" "Mit EES vergleichen" {
          tunnel: w386 -> [_ w626]
          frame False {
            n116 = property class="Arr (strict)"("Visible"=FALSE) -> ()  [unwired: 2 in, 2 out]
          }
          frame True {
            # "K->C°"
            # "Toleranz"
            n117 = call-poly <vilib>:"Read Delimited Spreadsheet.vi"("file path (dialog if empty)"=path "Z:/HT-Waermepumpe/Projekte/SubVi_EES_vergleich/test.txt", "format (%.3f)"="%,;%.3f") -> ("first row"=w633:dbl[])  [unwired: 8 in, 5 out]
            n118 = Delete From Array(array=w633, length=20) -> (deleted portion=w629:dbl[], array with subset deleted=w631:dbl[])  [unwired: 1 in]
            n119 = expression code="x-273.15"(w631) -> (w630:dbl[])
            n120 = Insert Into Array(array=string[] ["T 01", "T 02", "T 04", "T 05", "T 06", "T 07", "T 08", "T 09", "T 10", "T 11", "T 12", "T 13", "T 14", "T 35", "T 36", "T 38", "T 39"] ("Array"), new element=string[] ["COP_Öl", "m_dot_ENT_W", "m_dot_LIQ", "m_dot_MIX", "m_dot_oil", "m_dot_VAP", "m_dot_RES_W", "p_HD", "P_KOMP", "p_ND", "P_PUMP_th", "P_KOMP_th", "Q_dot_ENT", "Q_dot_ENT_W", "Q_dot_oil", "Q_dot_RES_W", "q_geg", "Q_dot_RES", "xi_LIQ", "xi_MIX"] ("Array")) -> (w640:string[])  [unwired: 1 in]
            n121 = property class="Arr (strict)"("Visible"=TRUE) -> ()  [unwired: 2 in, 2 out]
            n122 = Insert Into Array(array=w630, new element=w629) -> (w627:dbl[])  [unwired: 1 in]
            n123 = expression code="x*0.05"(w627) -> (w628:dbl[])
            n124 = Add(x=w627, y=w628) -> (x+y=w636:dbl[])
            n125 = Subtract(x=w627, y=w628) -> (x-y=w635:dbl[])
            n126 = Greater Or Equal?(x=w636, y=w626) -> (x >= y?=w637:bool[])
            n127 = Less Or Equal?(x=w635, y=w626) -> (x <= y?=w638:bool[])
            n128 = And(x=w637, y=w638) -> (x .and. y?=w634:bool[])
            n129 = Build Cluster Array(w627, w626, w640, w634) -> (→"?":T14)
          }
        }
        n130 = Index Array(array=w183, index #1=2 ("index"), index #2=3 ("index"), index #3=4, index #4=5, index #5=11 ("index")) -> (element #1=w250:dbl, element #2=w249:dbl, element #3=w248:dbl, element #4=w254:dbl, element #5=w231:dbl)
        n131 = Build Array(w250, w249, w248) -> (w247:dbl[])
        n132 = Index Array(array=w126, index #1=19, index #2=w371, index #3=w366, index #4=23) -> (element #1=w363:dbl, element #2=w362:dbl, element #3=w361:dbl, element #4=w360:dbl)
        n133 = Index Array(array=w183, index #1=w371, index #2=w366) -> (element #1=w369:dbl, element #2=w368:dbl)
        n134 = Array Max & Min(array=w247) -> (min value=w146:dbl)  [unwired: 3 out]
        n135 = call "Filter5"("Signal"=w368) -> ("Filtered Signal"=w364:dynamicdata)  [unwired: 9 in, 1 out]
        n136 = call "Filter4"("Signal"=w369) -> ("Filtered Signal"=w365:dynamicdata)  [unwired: 9 in, 1 out]
        n137 = Less?(x=w146, y=20.5 ("x")) -> (x < y?=w145:bool)
        n138 = Greater Or Equal?(x=w146, y=18.5 ("x")) -> (x >= y?=→"Druckzustand":bool)
        n139 = call "Convert from Dynamic Data11"("Dynamic Data Type"=w365) -> ("Scalar"=w359:dbl)  [unwired: 3 in]
        n140 = call "Convert from Dynamic Data12"("Dynamic Data Type"=w364) -> ("Scalar"=w358:dbl)  [unwired: 3 in]
        n141 = formula code="float32 TIM1; float32 P; float32 H; float32 K;\nH=0; K=0;\nTIM1=((TI36*FI35)+(TI32*FIOel))/(FI35+FIOel);\nif((TI36-TI35) > 2) {\nif((TIM1-TI35) < (0.2)) {\nH=1;}\nelse {\nH=0;}\nif((TI35-TI30) < (0.2)) {\nK=1;}\nelse {\nK=0; }\nP=100/(TIM1-TI30)*(TI35-TI30);\n}"("TI30"=w363, "TI32"=w362, "TI35"=w361, "TI36"=w360, "FIOel"=w359, "FI35"=w358) -> ("H"=w357:sgl, "K"=w354:sgl, "P"=→"%":sgl)  [unwired: 1 out]
        n142 = feedback #1() -> (w137:dbl)  [unwired: 1 in]
        n143 = Select(t=w128, s=w145, f=w137) -> (s? t:f=w138:dbl)
        n144 = feedback-in #1(w138) -> ()
        n145 = case shown="True" "Pumpen-Auto-Abschalt" {
          tunnel: w231 -> [_ w647]
          frame False {
          }
          frame True {
            n146 = Less?(x=w647, y=0.3) -> (x < y?=w646:bool)
            n147 = case shown="True" w646 {
              frame False {
              }
              frame True {
                n148 = local write "Pumpensteuerung"(0.0) -> ()
              }
            }
          }
        }
        n149 = Subtract(x=w128, y=w138) -> (x-y=w144:dbl)
        n150 = Greater Or Equal?(x=w254, y=9.9 ("x")) -> (x >= y?=w258:bool)
        n151 = Greater Or Equal?(x=w144, y=w143) -> (x >= y?=w142:bool)
        n152 = Or(x=w142, y=w258) -> (x .or. y?=w240:bool)
        n153 = Or(x="Drehzahl Bestätigung", y=w240) -> (x .or. y?=w242:bool)
        n154 = Equal?(x=w357, y=w353) -> (x = y?=→"warm":bool)
        n155 = Equal?(x=w354, y=w353) -> (x = y?=→"kalt":bool)
        n156 = feedback #2() -> (w241:dbl)  [unwired: 1 in]
        "Check" <- w241
        n157 = case shown="True" w240 {
          tunnel: w241 -> [w471 w475]
          tunnel: [w471 w476] -> w150
          frame False {
          }
          frame True {
            n158 = local write "Drehzahl SW"(1000.0) -> ()
            n159 = Multiply(x=w475, y=0.0) -> (x*y=w476:dbl)
            n160 = local write "Regler Hochdruck"(FALSE ("Regler Hochdruck")) -> ()
            n161 = local write "Exp.V"(60.0 ("Exp.V")) -> ()
          }
        }
        n162 = Select(t=0.0, s=w240, f="Drehzahl SW") -> (s? t:f=w244:dbl)
        n163 = feedback-in #2(w244, w242) -> ()
        n164 = local read "Konzentration"() -> (w124:dbl)
        n165 = case shown="True" "Rampe" {
          tunnel: [w427 w428] -> w149
          tunnel: w150 -> [w427 w430]
          frame False {
          }
          frame True {
            n166 = local read "Drehzahl"() -> (w429:dbl)
            n167 = formula code="if (ns > 100) {\nns=100;}\nif (ns < 1) {\nns=1;}\nif ((nSW>nSWR) &&  (nIW>=1000)) {\nnSWR=nSWR+ns;}\nelse {\nnSWR=nSW;}"("nSW"=w430, "ns"="Rampe rpm/s", "nIW"=w429) -> ("nSWR"=w428:dbl)
            "Rampe IW" <- w428
          }
        }
        n168 = case shown="True" "Xi / p_liq berechnung an" {
          tunnel: w126 -> [_ w470]
          tunnel: w183 -> [_ w463]
          tunnel: [0.0 w456] -> w233
          tunnel: [0.0 w453] -> w223
          tunnel: w125 -> [_ w451]
          tunnel: w124 -> [_ w450]
          frame False {
          }
          frame True {
            n169 = Index Array(array=w451, index=8) -> ()  [unwired: 1 out]
            n170 = Index Array(array=w463, index #1=4 ("index"), index #2=8 ("index")) -> (element #1=w458:dbl, element #2=w457:dbl)
            n171 = Index Array(array=w470, index #1=7 ("index"), index #2=6 ("index"), index #3=13 ("index"), index #4=14 ("index"), index #5=5 ("index")) -> (element #1=w462:dbl, element #2=w461:dbl, element #3=w460:dbl, element #4=w459:dbl, element #5=w454:dbl)
            n172 = script code="xi_a = xi_a/100;\ntry\nF = @(xi_r) ((refpropm('H','T',T6a+273.15,'P',p7*100,'ammonia','water',[xi_r 1-xi_r])*0.001-refpropm('H','T',T7+273.15,'P',p7*100,'ammonia','water',[xi_r 1-xi_r])*0.001)/(refpropm('H','T',T14+273.15,'P',p14*100,'ammonia','water',[xi_a 1-xi_a])*0.001-refpropm('H','T',T13+273.15,'P',p14*100,'ammonia','water',[xi_a 1-xi_a])*0.001)*(xi_a-1)+1-xi_r);\nxi_r0=xi_a;\n[xi_r, fval] = fzero(F,xi_r0);\n\np_liq=refpropm('P','T',T6+273.15,'Q',0,'ammonia','water',[xi_r 1-xi_r])/100;\ncatch\nxi_r=1\np_liq=refpropm('P','T',T6+273.15,'Q',0,'ammonia','water',[xi_r 1-xi_r])/100;\nend"("T7"=w462, "T6a"=w461, "T13"=w460, "T14"=w459, "xi_a"=w450, "p7"=w458, "p14"=w457, "T6"=w454) -> ("xi_r"=w456:dbl, "p_liq"=w453:dbl)  [unwired: 1 in, 1 out]
          }
        }
        "xi_r" <- w233
        "p_liq" <- w223
        n173 = Index Array(array=w183, index=13) -> (element=w185:dbl)
        n174 = Index Array(array=w126, index #1=18 ("index"), index #2=1 ("index"), index #3=22) -> (element #1=w115:dbl, element #2=w114:dbl, element #3=w116:dbl)
        n175 = call "Filter9"("Signal"=w223) -> ("Filtered Signal"=w221:dynamicdata)  [unwired: 9 in, 1 out]
        "p_liq_mittel" <- w221
        n176 = call "max_regelung.vi"("TI 21a IW °C"=w115, "TI 21a SW °C"="TI 21a SW °C", "Öl-Regelung"="Öl-Regelung", "TI 02 IW °C"=w114) -> ("zu"=w112:bool, "auf"=w113:bool)  [unwired: 6 in]
        "RV 30 auf" <- w113
        "RV 30 zu" <- w112
        n177 = call "Pumpensteuerung_PID.vi"("reinitialize? (F)"="reinitialize Pumpe", "PID Regelung Pumpe"="PID Regelung Pumpe", "FI13 SW in l/min"="FI13 SW in l/min", "Prozessvariable"=w185, "Pumpensteuerung"="Pumpensteuerung") -> ("upper limit"=w228:dbl)  [unwired: 4 in, 2 out]
        n178 = call "Senkenregler_PID.vi"("Regelventil 36"="Regelventil 36", "Solltemp."="TI35 SW", "Regelventil 35"="Regelventil 35", "Regler Senke"="Regler Senke", "reinitialize?"="reinitialize Senke", "TI_35"=w116) -> ("upper limit 2"=w237:dbl, "upper limit"=w235:dbl)  [unwired: 6 in, 2 out]
        n179 = Greater?(x=w221, y=15.0) -> (0:w220:dynamicdata)
        n180 = case shown="True" w220 {
          tunnel: [w442 15.0 ("y")] -> w219
          tunnel: w220 -> [w442 _]
          frame False {
          }
          frame True {
          }
        }
        n181 = call "Filter7"("Signal"=w228) -> ("Filtered Signal"=w227:dynamicdata)  [unwired: 9 in, 1 out]
        "Mittelwert" <- w227
        n182 = Add(x="zusätzlicher Druck", y=w219) -> (x+y=w218:dynamicdata)
        n183 = case shown="True" "Mittelwert Pumpe" {
          tunnel: w228 -> [w446 _]
          tunnel: [w446 w447] -> w229
          tunnel: w227 -> [_ w447]
          frame False {
          }
          frame True {
          }
        }
        n184 = Greater Than 0?(x="RV 33") -> (x > 0?=w262:bool)
        n185 = Less Than 0?(x="RV 33") -> (x < 0?=w261:bool)
        n186 = Select(t=w397, s=w261, f=w398) -> (s? t:f=w395:i32)
        n187 = Select(t=w397, s=w262, f=w398) -> (s? t:f=w396:i32)
        n188 = call "Hochdruckregler_PID.vi"("Regler Hochdruck"="Regler Hochdruck", "Steuereingang"=w218, "Solldruck"="PI05 SW", "PI05"=w183, "Exp.V"="Exp.V", "reinitialize? (F) in"="reinitialize HD") -> ("upper limit out"=w160:dbl)  [unwired: 7 in, 2 out]
        n189 = call "Filter8"("Signal"=w160) -> ("Filtered Signal"=w224:dynamicdata)  [unwired: 9 in, 1 out]
        "Mittelwert 2" <- w224
        n190 = case shown="True" "Mittelwert HD" {
          tunnel: w160 -> [w444 _]
          tunnel: [w444 w445] -> w225
          tunnel: w224 -> [_ w445]
          frame False {
          }
          frame True {
          }
        }
        n191 = call "Stellungen_Namen2.vi"("Kühlventil"=w237, "Pumpensteuerung"=w229, "Regelventil 39"="Regelventil 39", "Exp.V"=w225, "Regelventil 14"=w235, "Meter"=w149, "zu"=w112, "auf"=w113, "Regelventil 34"="Regelventil 34") -> ("Dynamic Data"=w293:dynamicdata)  [unwired: 2 in]
        n192 = Build Array("PI05 SW", "TI35 SW", "FI13 SW in l/min") -> (w156:dbl[])
        n193 = Merge Signals(w293, w396, w395) -> (w161:dynamicdata)
        n194 = Insert Into Array(array=w125, new element=w156) -> (w127:dbl[])  [unwired: 1 in]
        n195 = call-poly <vilib>:"DAQmx Write.vi"("task/channels in"=w163, "auto start"=w164, "data"=w161, "error in"=w162) -> ()  [unwired: 9 in, 3 out]
        n196 = Index Array(array=w126, index=18) -> (element=w285:dbl)
        n197 = Index Array(array=w183, index #1=1, index #2=0, index #3=7, index #4=6) -> (element #1=w282:dbl, element #2=w281:dbl, element #3=w280:dbl, element #4=w279:dbl)
        n198 = Index Array(array=w127, index=0) -> (element=w216:dbl)
        n199 = Not Equal To 0?(x=w216) -> (x != 0?=w136:bool)
        n200 = Divide(x=w282, y=w281) -> (x/y=w403:dbl)
        "Druckverhältnis" <- w403
        n201 = Subtract(x=w280, y=w279) -> (x-y=w413:dbl)
        n202 = Greater?(x=w413, y=1.0) -> (0:w287:bool)
        "Fl.Pumpe an" <- w287
        n203 = feedback #3() -> (w134:dbl)  [unwired: 1 in]
        n204 = Select(t=w134, s=w136, f=w128) -> (s? t:f=w135:dbl)
        n205 = feedback-in #3(w135) -> ()
        n206 = Less?(x=w285, y=60) -> (x < y?=w349:bool)
        "Temperatur Öl" <- w349
        n207 = Greater?(x=w403, y=1.5) -> (0:w401:bool)
        n208 = feedback #4(w128) -> (w129:dbl)
        n209 = Select(t=w128, s="Reset", f=w129) -> (s? t:f=w130:dbl)
        n210 = feedback-in #4(w130) -> ()
        n211 = Subtract(x=w128, y=w135) -> (x-y=w133:dbl)
        n212 = Subtract(x=w128, y=w130) -> (x-y=w132:dbl)
        n213 = expression code="x-3600"(w133) -> (w406:dbl)
        n214 = Build Array(w349, w401) -> (→"Warnungen":bool[])
        n215 = expression code="x-3600"(w132) -> (w408:dbl)
        n216 = Greater?(x=w133, y=630.0) -> (0:w288:bool)
        "Magnetventil" <- w288
        n217 = Build Array(w136, w288, w287) -> (→"Status Komponenten":bool[])
        n218 = call "Verdichternamen.vi"("Array"=w127) -> ("Dynamic Data"=w404:dynamicdata)  [unwired: 10 in]
        n219 = Seconds To Date/Time(time stamp (now)=w406) -> (date time rec=w350:T15)  [unwired: 1 in]
        n220 = Seconds To Date/Time(time stamp (now)=w408) -> (date time rec=w417:T15)  [unwired: 1 in]
        n221 = Unbundle By Name(w417) -> ("second"=w416:i32, "minute"=w415:i32, "hour"=w409:i32)
        n222 = Unbundle By Name(w350) -> ("second"=w419:i32, "minute"=w418:i32, "hour"=w407:i32)
        n223 = Bundle("second"=w419, "minute"=w418, "hour"=w407) -> (→"Verdichteraktivität":cluster{"second":i32, "minute":i32, "hour":i32})  [unwired: 1 in]
        n224 = Bundle("second"=w416, "minute"=w415, "hour"=w409) -> (→"Betriebszeit":cluster{"second":i32, "minute":i32, "hour":i32})  [unwired: 1 in]
        n225 = local read "Array 2"() -> (w122:waveform(dbl)[])
        n226 = Merge Signals(w178, w177, w293, w404, w122) -> (w312:dynamicdata)
        n227 = flat-sequence {
          tunnel: [w505] -> w426
          tunnel: [w504] -> w425
          tunnel: w330 -> [w503]
          tunnel: w329 -> [w502]
          tunnel: [w500] -> w326
          tunnel: "Identität!" -> [w499]
          tunnel: "Dateiname!" -> [w498]
          tunnel: "Speichern" -> [w497]
          tunnel: "tag" -> [w496]
          tunnel: w426 -> [w603]
          tunnel: w425 -> [w602]
          tunnel: [w598] -> w333
          tunnel: [w600] -> w332
          tunnel: w331 -> [w599]
          frame #0 {
            n228 = Index Array(array=w502) -> (element=w501:timestamp)  [unwired: 1 in]
            n229 = event shown="[1] \"Speichern\": Value Change" {
              selector: _ -> [_ _ _]
              dyn-events: _ -> [_ _ _]
              timeout: 5 -> [_ _ _]
              tunnel: [_ w515 _] -> w505
              tunnel: w503 -> [_ w510 _]
              tunnel: ["" w514 ""] -> w504
              tunnel: w501 -> [_ w513 w584]
              tunnel: [_ _ w582] -> w500
              tunnel: w499 -> [_ w512 _]
              tunnel: w498 -> [_ w511 _]
              tunnel: w497 -> [_ w509 _]
              tunnel: w496 -> [_ w508 _]
              event Timeout {
                n230 = event-data() -> ()  [unwired: 1 in, 1 out]
              }
              event "Speichern": Value Change {
                n231 = event-data() -> ()  [unwired: 1 in, 1 out]
                n232 = case shown="False" w509 {
                  tunnel: [w547 _] -> w515
                  tunnel: [w542 _] -> w514
                  tunnel: w513 -> [w534 _]
                  tunnel: w512 -> [w518 _]
                  tunnel: w511 -> [w530 _]
                  tunnel: w510 -> [w529 _]
                  tunnel: w508 -> [w517 _]
                  frame False {
                    w521 = "\r"
                    n233 = property on="Dateiname!" class="Str"("DisabledEnum"=T4."Disabled and Grayed Out" ("Disabled")) -> ()  [unwired: 2 in, 2 out]
                    n234 = for {
                      N: 1 -> [_]
                      tunnel: ["Zeit"] -> w527 mode=indexing
                      tunnel: ["Kommentar"] -> w523 mode=indexing
                    }
                    n235 = Format Date/Time String(time format string (%c)="%d-%m-%Y_%H.%M ", seconds (now)=w534) -> (date/time string=w535:string)  [unwired: 1 in]
                    n236 = Concatenate Strings(w518, "\\", w535, w530, ".lvm" ("string")) -> (w537:string)
                    n237 = Insert Into Array(array=w529, index (row)=0, new element=w527) -> (w525:string[][])  [unwired: 1 in]
                    n238 = Build Path(base path=path "\\\\pcift88\\Studenten/HT-Waermepumpe/Messdaten" ("file path (dialog if empty)"), name or relative path=w537) -> (appended path=w532:path)
                    n239 = Concatenate Strings(w518, "\t", "tag: " ("string"), w517) -> (w516:string)
                    n240 = Insert Into Array(array=w525, new element=w523) -> (w524:string[][])  [unwired: 2 in]
                    n241 = Open/Create/Replace File(file path (use dialog)=w532, operation (0:open)=T11."replace or create with confirmation") -> (refnum out=→"refnum out":refnum<file>, error out=w547:errorcluster)  [unwired: 4 in, 1 out]
                    n242 = Transpose 2D Array(2D array=w524) -> (transposed array=w545:string[][])
                    n243 = Format Date/Time String(seconds (now)=w534) -> (date/time string=w544:string)  [unwired: 2 in]
                    n244 = Strip Path(path=w532) -> (name=w531:string)  [unwired: 1 out]
                    n245 = Array To Spreadsheet String(array=w545, 3:"%s" ("format string")) -> (spreadsheet string=w543:string)  [unwired: 1 in]
                    n246 = Concatenate Strings(w516, w521, w521, w531, w521, w521, w544, w521, w521, w543, w521, w521) -> (w542:string)
                  }
                  frame True {
                    n247 = local read "refnum out"() -> (w551:refnum<file>)
                    n248 = property on="Dateiname!" class="Str"("DisabledEnum"=T4."Enabled" ("Disabled")) -> ()  [unwired: 2 in, 2 out]
                    n249 = Close File(refnum=w551) -> ()  [unwired: 1 in, 2 out]
                  }
                }
              }
              event "Comment": Value Change {
                # "Umlaute + ß ersetzen, quick&dirty 4.1.2016"
                n250 = event-data() -> ()  [unwired: 1 in, 1 out]
                n251 = flat-sequence {
                  tunnel: ["Kommentar"] -> w552
                  tunnel: w584 -> [w588]
                  frame #0 {
                    w590 = "\r"
                    n252 = local read "Historie"() -> (w592:string)
                    n253 = Get Date/Time String(seconds (now)=w588, want seconds? (F)=TRUE) -> (time string=w591:string)  [unwired: 1 in, 1 out]
                    n254 = Concatenate Strings(w592, w591, " -> ", "Kommentar", w590, w590) -> (→"Historie":string)
                  }
                  frame #1 {
                    n255 = local write "Kommentar"("") -> ()
                  }
                }
                n256 = Search and Replace String(replace all?=TRUE, input string=w552, search string="ä", replace string="ae") -> (result string=w574:string)  [unwired: 4 in, 3 out]
                n257 = Search and Replace String(replace all?=TRUE, input string=w574, search string="ü", replace string="ue") -> (result string=w573:string)  [unwired: 4 in, 3 out]
                n258 = Search and Replace String(replace all?=TRUE, input string=w573, search string="ö", replace string="oe") -> (result string=w572:string)  [unwired: 4 in, 3 out]
                n259 = Search and Replace String(replace all?=TRUE, input string=w572, search string="ß", replace string="ss") -> (result string=w553:string)  [unwired: 4 in, 3 out]
                n260 = Search and Replace String(replace all?=TRUE, input string=w553, search string="Ä", replace string="Ae") -> (result string=w562:string)  [unwired: 4 in, 3 out]
                n261 = Search and Replace String(replace all?=TRUE, input string=w562, search string="Ü", replace string="Ue") -> (result string=w561:string)  [unwired: 4 in, 3 out]
                n262 = Search and Replace String(replace all?=TRUE, input string=w561, search string="Ö", replace string="Oe") -> (result string=w554:string)  [unwired: 4 in, 3 out]
                n263 = for {
                  N: 1 -> [_]
                  tunnel: [w585] -> w582 mode=indexing
                  tunnel: w554 -> [w585]
                }
              }
            }
          }
          frame #1 {
            n264 = local read "refnum out"() -> (w595:refnum<file>)
            n265 = Concatenate Strings(w602, w599) -> (w601:string)
            n266 = Not A Number/Path/Refnum?(number/path/refnum=w595) -> (NaN/Path/Refnum?=w596:bool)
            n267 = Set File Position(refnum=w595, from (0:start)=enum16{"start", "end", "current"}."end", error in=w603) -> (refnum out=w604:refnum<file>, error out=w605:errorcluster)  [unwired: 1 in]
            n268 = Not(x=w596) -> (.not. x?=→"Speichert!":bool)
            n269 = Write to Text File(file (use dialog)=w604, text=w601, error in=w605) -> (refnum out=w598:refnum<file>, error out=w600:errorcluster)  [unwired: 1 in, 1 out]
          }
        }
        n270 = Empty String/Path?(string/path="Identität!") -> (empty?=w324:bool)
        n271 = Empty String/Path?(string/path="Dateiname!") -> (empty?=w323:bool)
        n272 = Or(x=w324, y=w323) -> (x .or. y?=w320:bool)
        n273 = call "Protokollordnung"("Signals"=w312) -> ("Signal Out"=w338:dynamicdata)  [unwired: 9 in, 1 out]
        n274 = Boolean To (0,1)(Boolean=w320) -> (0, 1=w321:i16)
        n275 = expression code="x*2"(w321) -> (w322:i16)
        n276 = property on="Speichern" class="Bool (strict)"("DisabledEnum"=w322) -> ()  [unwired: 2 in, 2 out]
        n277 = call "Convert from Dynamic Data"("Dynamic Data Type"=w338) -> ("Array of Waveform"=w339:waveform(dbl)[])  [unwired: 3 in]
        n278 = Array Size(array=w339) -> (size(s)=w316:i32)
        n279 = Concatenate Strings("%" ("string"), "." ("string"), ";%g" ("string")) -> (w341:string)
        n280 = Initialize Array(w341, w316) -> (w340:string[])
        n281 = for {
          tunnel: w339 -> [w609] mode=indexing
          tunnel: [w616] -> w336 mode=indexing
          tunnel: w340 -> [w614] mode=indexing
          tunnel: [w608] -> w330 mode=indexing
          tunnel: [w610] -> w329 mode=indexing
          tunnel: [w611] -> w335 mode=indexing
          n282 = Unbundle By Name(w609) -> ("Y"=w615:dbl[], "t0"=w607:timestamp)
          n283 = Get Waveform Attribute(5:w607, 6:"NI_ExpTimeStamp", 7:w609) -> (1:w610:timestamp)  [unwired: 1 in, 3 out]
          n284 = for {
            tunnel: w615 -> [w623] mode=indexing
            tunnel: [w622] -> w616 mode=indexing
            tunnel: w614 -> [w621]
            tunnel: w609 -> [w620]
            tunnel: [w619] -> w608 mode=indexing
            n285 = Format Into String(format string=w621, w623) -> (resulting string=w622:string)  [unwired: 2 in, 1 out]
            n286 = Get Waveform Attribute(5:"", 6:"NI_ChannelName", 7:w620) -> (1:w619:string)  [unwired: 1 in, 3 out]
          }
          n287 = Format Date/Time String(time format string (%c)="%H.%M.%S", seconds (now)=w610) -> (date/time string=w611:string)  [unwired: 1 in]
        }
        n288 = Insert Into Array(array=w336, index (row)=0, new element=w335) -> (w327:string[][])  [unwired: 1 in]
        n289 = Increment(x=w316) -> (x+1=w317:i32)
        n290 = Insert Into Array(array=w327, index (row)=w317, new element=w326) -> (w328:string[][])  [unwired: 1 in]
        n291 = Transpose 2D Array(2D array=w328) -> (transposed array=w325:string[][])
        n292 = Array To Spreadsheet String(array=w325, 3:"%s" ("format string")) -> (spreadsheet string=w331:string)  [unwired: 1 in]
      }
      frame #2 {
        n293 = Tick Count (ms)() -> (millisecond timer value=w741:u32)
        n294 = Subtract(x=w741, y=w740) -> (x-y=w739:u32)
        n295 = Divide(x=w739, y=1000.0) -> (x/y=→"Schleifendauer":dbl)
      }
    }
  }
  n296 = while {
    tunnel: w4 -> [w748]
    tunnel: w3 -> [w747]
    tunnel: w7 -> [w746]
    stop <- w745 stop-if-true
    n297 = case shown="True" "Keithley Messung?" {
      tunnel: w748 -> [_ w758]
      tunnel: w747 -> [_ w757]
      tunnel: w746 -> [_ w756]
      tunnel: [w749 w753] -> w745
      frame False {
        n298 = local read "Programm stoppen!"() -> (w749:bool)
      }
      frame True {
        n299 = flat-sequence {
          tunnel: [w788] -> w780
          tunnel: w757 -> [w785]
          tunnel: [w790] -> w779
          tunnel: w756 -> [w788]
          tunnel: w758 -> [w789]
          tunnel: [w784] -> w778
          tunnel: w780 -> [w794]
          tunnel: [w794] -> w777
          tunnel: [w793] -> w776
          tunnel: w779 -> [w793]
          tunnel: w778 -> [w792]
          tunnel: [w792] -> w775
          tunnel: w777 -> [w798]
          tunnel: [w798] -> w774
          tunnel: w776 -> [w800]
          tunnel: [w799] -> w773
          tunnel: [w797] -> w772
          tunnel: w775 -> [w796]
          tunnel: w774 -> [w804]
          tunnel: [w804] -> w771
          tunnel: w773 -> [w803]
          tunnel: [w803] -> w770
          tunnel: [w802] -> w769
          tunnel: w772 -> [w802]
          tunnel: w771 -> [w807]
          tunnel: [w807] -> w768
          tunnel: [w811] -> w767
          tunnel: [w810] -> w766
          tunnel: [w809] -> w765
          tunnel: w770 -> [w806]
          tunnel: w769 -> [w805]
          tunnel: w768 -> [w817]
          tunnel: [w816] -> w751
          tunnel: w767 -> [w815]
          tunnel: w766 -> [w814]
          tunnel: w765 -> [w818]
          tunnel: [w815] -> w760
          tunnel: [w814] -> w759
          frame #0 {
            n300 = Format Into String(format string="%.0f", w788) -> (resulting string=w783:string)  [unwired: 2 in, 1 out]
            n301 = Concatenate Strings("TRAC:CLE:AUTO ON\nTRAC:POIN ", w783, "\nTRAC:FEED SENS\nTRAC:FEED:CONT NEXT\nINIT\n" ("Daten")) -> (w781:string)
            n302 = VISA Write(VISA resource name=w789, write buffer=w781, error in (no error)=w785) -> (VISA resource name out=w790:refnum<visa-resource-name>, error out=w784:errorcluster)  [unwired: 1 out]
          }
          frame #1 {
            (unwired) u32 1600 ("ms Wartezeit")
            n303 = Wait (ms)(milliseconds to wait="Wartezeit 1") -> ()  [unwired: 1 out]
          }
          frame #2 {
            n304 = VISA Write(VISA resource name=w800, write buffer="FORM:ELEM READ\nTRAC:DATA?\n", error in (no error)=w796) -> (VISA resource name out=w799:refnum<visa-resource-name>, error out=w797:errorcluster)  [unwired: 1 out]
          }
          frame #3 {
            (unwired) u32 200 ("ms Wartezeit")
            n305 = Wait (ms)(milliseconds to wait="Wartezeit 2") -> ()  [unwired: 1 out]
          }
          frame #4 {
            n306 = property class="Instr"(reference=w806, error in=w805) -> (reference out=w812:refnum<visa-resource-name>, error out=w813:errorcluster, "Bytes at Port"=w808:u32)
            n307 = VISA Read(VISA resource name=w812, byte count=w808, error in (no error)=w813) -> (VISA resource name out=w811:refnum<visa-resource-name>, read buffer=w809:string, error out=w810:errorcluster)  [unwired: 1 out]
          }
          frame #5 {
            n308 = Initialize Array(0.0 ("Elementdaten"), w817) -> (w823:dbl[])
            n309 = Concatenate Strings(w818, "," ("Sub-Sring")) -> (w820:string)
            n310 = for {
              N: w817 -> [_]
              shift-right: [w833] -> w816
              shift-left: w823 -> [w824]
              shift-right: [w826] -> _
              shift-left: w820 -> [w832]
              shift-right: [w827] -> _
              shift-left: 0 -> [w828]
              n311 = Increment(x=w828) -> (x+1=w827:i32)
              n312 = Match Pattern(string=w832, regular expression="," ("gültiger Ausdruck")) -> (before substring=w829:string, after substring=w826:string)  [unwired: 1 in, 2 out]
              n313 = Fract/Exp String To Number(use system decimal point (T)=FALSE ("verwende System-Dezimalpunkt (T)"), string=w829) -> (number=w830:dbl)  [unwired: 2 in, 1 out]
              n314 = Replace Array Subset(array=w824, new element=w830, index=w828) -> (w833:dbl[])
            }
          }
        }
        n315 = VISA Close(VISA resource name=w760, error in (no error)=w759) -> ()  [unwired: 1 out]
        n316 = formula code="a[1]=a[1]*1.01004457922915+0.133068086896257;\na[2]=a[2]*1.01014117233966+0.294180417452684;\na[3]=a[3]*1.00993637757344+0.209441824398475;\na[4]=a[4]*1.00932973010682+0.259262926047991;\na[5]=a[5]*1.00930331568572+0.228927332490957;\na[6]=a[6]*1.01024538439511+0.201727412078399;\na[7]=a[7]*1.0087269878036+0.197454569443902;\na[8]=a[8]*1.00817958579574+0.231348275618626;\na[9]=a[9]*1.00724396151288+0.241229434064865;\na[10]=a[10]*1.00682889774394+0.351755663965879;\na[11]=a[11]*1.00976696877551+0.333892118677183;\na[12]=a[12]*1.00865305218374+0.233585111220767;\na[13]=a[13]*1.00773724644154+0.244161339419892;\na[14]=a[14]*1.00732094954563+0.266813493780242;\na[15]=a[15]*1.00948724024148+0.279354562608908;\na[16]=a[16]*1.01022977309037+0.392758213231019;\na[17]=a[17]*1.01097708318306+0.272598351778253;\na[18]=a[18]*1.01024985874356+0.31466479050415;\na[19]=a[19]*1.01027646591523+0.294875486610268;\na[20]=a[20]*1.01100669138143+0.279515685632888;\na[21]=a[21]*1.00981092377617+0.0578953355238254;\na[22]=a[22]*1.00991834209257+-0.011277611587031;\na[23]=a[23]*1.01126977561923+0.141506604757659;\na[24]=a[24]*10.472210659+20.86592732;\na[25]=a[25]*1.01025466547592+0.0497908086538084;\na[26]=a[26]*1.00976426773433+0.220308523877263;\na[27]=a[27]*1.00903110633516+0.245963622913526;\na[28]=a[28]*1.0093732830457+0.22956222955169;\na[29]=a[29]*1.00801044196409+0.264174857336899;\na[30]=a[30]*10.472210659+20.86592732;\na[31]=a[31]*0.999393990507397+0.191440503754075;\na[32]=a[32]*0.999373205846434+0.328535587481704;\na[33]=a[33]*-7.81768921988146E-37+117.519821341696;\na[34]=a[34]*1.00361983406042+-0.0692074273728668;\na[35]=a[35]*1.00636292098329+0.244799017162493;\na[36]=a[36]*1.00330761644872+0.293678462611463;\na[37]=a[37]*1.00374954586531+0.130221452629569;\na[38]=a[38]*1.00364681107463+0.216241713634085;\na[39]=a[39]*0.997695329703211+0.265834404714938;\na[40]=a[40]*0+0;\na[41]=a[41]*1.00136234738459+0.128728737281737;\na[42]=a[42]*1.00211548380731+0.11138737377543;\na[43]=a[43]*1.00267060229531+0.0240889679585784;\na[44]=a[44]*1.00251334553129+0.0553082853626103;\na[45]=a[45]*1.00252085185119+0.0647890721242934;\na[46]=a[46]*1.00225534085789+0.0690565724320581;\na[47]=a[47]*1.00301151320947+0.0270509161078601;\na[48]=a[48]*-2.02711381500172+59.3046192294426;\na[49]=a[49]*1.00734414716346+-0.121350482921622;\na[50]=a[50]*1.00592015374179+-0.0634948677207755;\na[51]=a[51]*1.01444217353956+-0.00252289638416766;\na[52]=a[52]*1.01340425941479+-0.0725471269515714;\na[53]=a[53]*1.01313501929496+-0.0458472582251906;\na[54]=a[54]*1.01441546629149+-0.0348099221920813;\na[55]=a[55]*1.01806506689285+-0.287608176723632;\na[56]=a[56]*1.00298391764093+0.0906055660902276;\na[57]=a[57]*1.00218268319988+0.127855155796493;\na[58]=a[58]*1.00424909966908+0.062050663126158;\na[59]=a[59]*1.00474010545054+0.0499038731954779;\na[60]=a[60]*1.00453848593804+0.0990108472166527;\na[61]=a[61]*1.00049616672594+0.06663475091954;\na[62]=a[62]*1.00353720447264+-0.148903551813917;\na[63]=a[63]*1.0013386704508+0.0703655146896246;\na[64]=a[64]*1.00176958087407+0.0712416169689185;\na[65]=a[65]*1.00615291190021+-0.0245847102131905;\na[66]=a[66]*1.00293906171594+0.0492894291585169;\na[67]=a[67]*1.00316510091213+0.0810115232132156;\na[68]=a[68]*1.00186368714515+0.101174937275108;\na[69]=a[69]*0.99911008843497+0.208022552658852;\na[70]=a[70]*1.00113678797085+0.0691400739377397;\na[71]=a[71]*1.00065440599176+-0.060014211713649;\na[72]=a[72]*0.999028733306485+0.162385101053749;\na[73]=a[73]*1.01415750602093+-0.153848802691124;\na[74]=a[74]*0.996846470632035+0.00904842968552529;\na[75]=a[75]*1.00329276661982+0.0980030220129681;\na[76]=a[76]*1.00305161992432+0.0636495588009406;\na[77]=a[77]*1.00188307513449+-0.0184147194045401;\na[78]=a[78]*1.00031415473799+0.119240353746171;\na[79]=a[79]*1.00238676505746+0.0609148545056717;\na[80]=a[80]*0+0;\na[81]=a[81]*1.00268890168907+0.146689737211891;\na[82]=a[82]*1.00524955707108+0.0880320569989309;\na[83]=a[83]*0.998910188712216+0.110706775173153;\na[84]=a[84]*0.999620856867206+0.0657807706063342;\na[85]=a[85]*0.999955063214442+0.0298200618116295;\na[86]=a[86]*1.00094407271355+0.00928621208674304;\na[87]=a[87]*1.00290719527849+-0.0153081923840468;\na[88]=a[88]*1.00058227563664+0.0478384916212647;\na[89]=a[89]*1.00012000903421+0.0614115295400301;\na[90]=a[90]*1.0013157102207+0.04814609252972;\na[91]=a[91]*3.85443755821328E-37+41.8149896833333;\na[92]=a[92]*1.0053509980059+-0.320538777367804;\na[93]=a[93]*1.00268428117572+-0.354260534572677;\na[94]=a[94]*1.00051023409583+-0.324175219439094;\na[95]=a[95]*0.998605102826142+-0.251781331971186;\na[96]=a[96]*0.99836145718677+-0.215356826219976;\na[97]=a[97]*0.999823175052141+-0.317432574540277;\na[98]=a[98]*0.999725313576774+-0.301039232969554;\na[99]=a[99]*1.00152827663098+-0.334554166873532;\na[100]=a[100]*0+0;\na[101]=a[101]*1.00380710958452+0.114544204126345;\na[102]=a[102]*1.00307092860053+0.0657296244616742;\na[103]=a[103]*1.00177097861115+0.0545355315993369;\na[104]=a[104]*1.00351917901712+0.0298830366875289;\na[105]=a[105]*1.00045555236917+0.0986724021942105;\na[106]=a[106]*1.00675343767772+0.041571292581132;\na[107]=a[107]*1.01591812136243+-0.181236061070024;\na[108]=a[108]*1.00874399369149+-0.0247944970277671;\na[109]=a[109]*1.00998086112529+-0.0381486120485471;\na[110]=a[110]*0+0;\na[111]=a[111]*0+0;\na[112]=a[112]*0+0;\na[113]=a[113]*0+0;\na[114]=a[114]*0+0;\na[115]=a[115]*0+0;\na[116]=a[116]*0+0;\na[117]=a[117]*0+0;\na[118]=a[118]*0+0;\na[119]=a[119]*0+0;\na[120]=a[120]*0+0;"("a"=w751) -> ("a"=w750:dbl[])
        n317 = call "Messplattenanzeige.vi"("Array"=w750) -> ()  [unwired: 11 in]
        n318 = Get Date/Time In Seconds() -> (seconds since 1Jan1904=w755:timestamp)
        n319 = Spreadsheet String To Array(delimiter (Tab)=",", format string="%.3f", spreadsheet string="TC 101,TC 102,TC 103,TC 104,TC 105,TC 106,TC 107,TC 108,TC 109,TC 110,TC 111,TC 112,TC 113,TC 114,TC 115,TC 116,TC 117,TC 118,TC 119,TC 120,TC 121,TC 122,TC 123,TC 124,TC 125,TC 126,TC 127,TC 128,TC 129,TC 130,TC 131,TC 132,TC 133,TC 134,TC 135,TC 136,TC 137,TC 138,TC 139,TC 140,TC 201,TC 202,TC 203,TC 204,TC 205,TC 206,TC 207,TC 208,TC 209,TC 210,TC 211,TC 212,TC 213,TC 214,TC 215,TC 216,TC 217,TC 218,TC 219,TC 220,TC 221,TC 222,TC 223,TC 224,TC 225,TC 226,TC 227,TC 228,TC 229,TC 230,TC 231,TC 232,TC 233,TC 234,TC 235,TC 236,TC 237,TC 238,TC 239,TC 240,TC 301,TC 302,TC 303,TC 304,TC 305,TC 306,TC 307,TC 308,TC 309,TC 310,TC 311,TC 312,TC 313,TC 314,TC 315,TC 316,TC 317,TC 318,TC 319,TC 320,TC 401,TC 402,TC 403,TC 404,TC 405,TC 406,TC 407,TC 408,TC 409,TC 410,TC 411,TC 412,TC 413,TC 414,TC 415,TC 416,TC 417,TC 418,TC 419,TC 420", array type (2D Dbl)=string[] []) -> (array=w763:string[])
        n320 = for {
          tunnel: w763 -> [w839] mode=indexing
          tunnel: [w836] -> w752 mode=indexing
          tunnel: w755 -> [w835]
          tunnel: w750 -> [w834] mode=indexing
          n321 = Build Array(w834) -> (w838:dbl[])
          n322 = Bundle By Name("Y"=w838, "t0"=w835) -> (w837:waveform(dbl))  [unwired: 1 in]
          n323 = Set Waveform Attribute(5:w839, 6:"NI_ChannelName", 7:w837) -> (3:w836:waveform(dbl))  [unwired: 1 in, 2 out]
        }
        "Array 2" <- w752
        n324 = local read "Programm stoppen!"() -> (w753:bool)
      }
    }
  }
  n325 = call <vilib>:"DAQmx Clear Task.vi"("task in"=w16, "error in"=w14) -> ()  [unwired: 13 in, 1 out]
  n326 = call <vilib>:"DAQmx Clear Task.vi"("task in"=w15, "error in"=w13) -> ()  [unwired: 13 in, 1 out]
  n327 = Close File(refnum=w41, error in=w40) -> (error out=w44:errorcluster)  [unwired: 1 out]
  n328 = call <vilib>:"General Error Handler.vi"("error in (no error)"=w44, "[exception action] (none:0)"=1 ("[exception code]"), "[exception code]"=1) -> ()  [unwired: 8 in, 5 out]
